vi "water-level (1).vi"() -> ()   [LabVIEW 2020]
panel:
  in  "Table Control":string[][](table)
  in  "VISA resource name":refnum<visa-resource-name>
  out "Tank":dbl(slide) scale=0.0..10.0
  out "water level low":bool
  out "water level high":bool
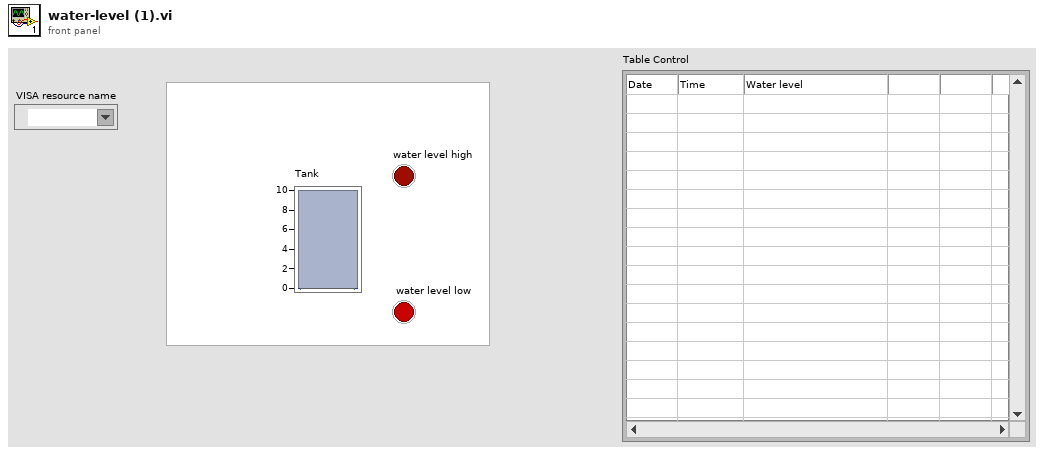
[diagram p1: front panel]
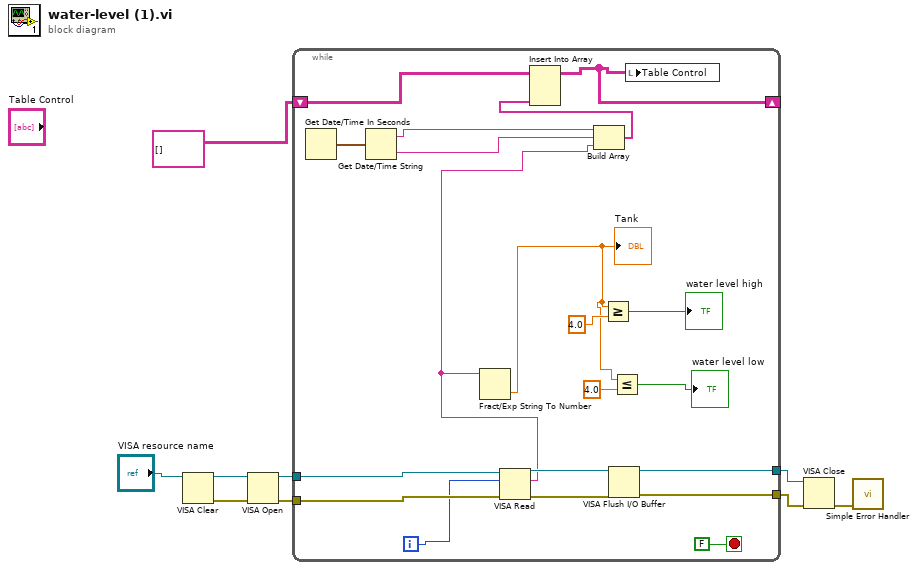
[diagram p0: block diagram]
diagram:
  n1 = VISA Clear(VISA resource name="VISA resource name") -> (VISA resource name out=w7:refnum<visa-resource-name>, error out=w8:errorcluster)  [unwired: 1 in]
  n2 = VISA Open(error in (no error)=w8, VISA resource name=w7) -> (VISA resource name=w6:refnum<visa-resource-name>, error out=w5:errorcluster)  [unwired: 3 in]
  n3 = while {
    tunnel: w6 -> [w24]
    tunnel: w5 -> [w23]
    tunnel: [w19] -> w2
    tunnel: [w18] -> w3
    shift-right: [w10] -> _
    shift-left: string[][] [] -> [w11]
    i -> [w22]
    stop <- FALSE stop-if-true
    n4 = Get Date/Time In Seconds() -> (seconds since 1Jan1904=w16:timestamp)
    n5 = Get Date/Time String(seconds (now)=w16) -> (date string=w15:string, time string=w14:string)  [unwired: 2 in]
    n6 = VISA Read(VISA resource name=w24, byte count=w22, error in (no error)=w23) -> (VISA resource name out=w21:refnum<visa-resource-name>, read buffer=w13:string, error out=w20:errorcluster)  [unwired: 1 out]
    n7 = Fract/Exp String To Number(string=w13) -> (number=w17:dbl)  [unwired: 3 in, 1 out]
    "Tank" <- w17
    n8 = Build Array(w15, w14, w13) -> (w12:string[])
    n9 = Insert Into Array(array=w11, new element=w12) -> (w10:string[][])  [unwired: 2 in]
    n10 = Greater Or Equal?(x=w17, y=4.0) -> (x >= y?=→"water level high":bool)
    n11 = VISA Flush I/O Buffer(VISA resource name=w21, error in (no error)=w20) -> (VISA resource name out=w18:refnum<visa-resource-name>, error out=w19:errorcluster)  [unwired: 1 in]
    n12 = Less Or Equal?(x=w17, y=4.0) -> (x <= y?=→"water level low":bool)
    n13 = local write "Table Control"(w10) -> ()
  }
  n14 = VISA Close(VISA resource name=w3, error in (no error)=w2) -> (error out=w4:errorcluster)
  n15 = call <vilib>:"Simple Error Handler.vi"("error in (no error)"=w4) -> ()  [unwired: 4 in, 5 out]
